vi "Analyze Data.vi"(0 "Weather Data":dynamicdata(waveform), 11 "error in":errorcluster) -> (4 "Time":dbl, 6 "Temperature":dbl, 8 "Wind Speed":dbl, 15 "error out":errorcluster)   [LabVIEW 2010]
uses:
  Instance           1 20Saved   Analyze Data .vi
  Instance           3 20Saved   Analyze Data .vi
  Instance           4 20Saved   Analyze Data .vi
  Instance           5 20Saved   Analyze Data .vi
  Instance           2 20Saved   Analyze Data .vi
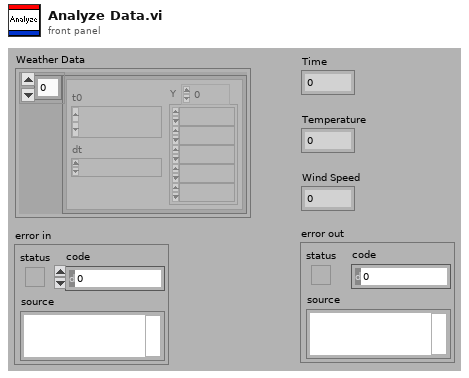
[diagram p1: front panel]
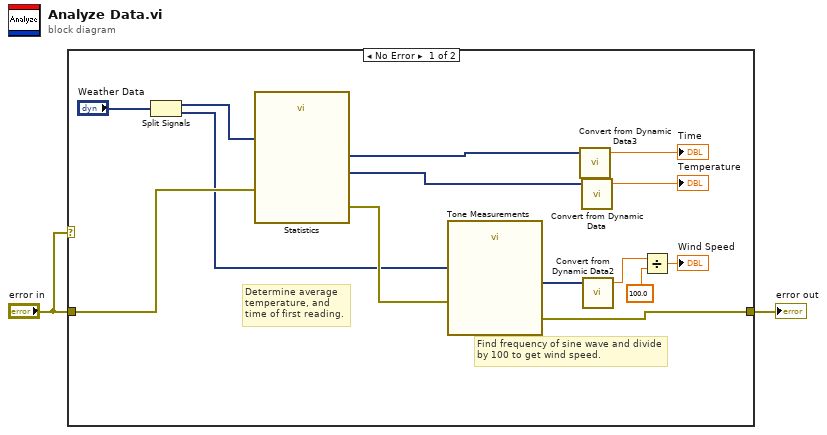
[diagram p0: block diagram]
diagram:
  n1 = case shown="No Error" "error in" {
    tunnel: "error in" -> [w16 w17]
    tunnel: [w10 w17] -> w2
    frame No Error {
      # "Find frequency of sine wave and divide by 100 to get wind speed."
      # "Determine average temperature, and time of first reading."
      n2 = Split Signals("Weather Data") -> (w4:dynamicdata, w3:dynamicdata)  [unwired: 2 in]
      n3 = call "Statistics"("Signals"=w4, "error in (no error)"=w16) -> ("Arithmetic Mean"=w5:dynamicdata, "First Time"=w11:dynamicdata, "error out"=w9:errorcluster)  [unwired: 23 in]
      n4 = call "Tone Measurements"("error in (no error)"=w9, "Signals"=w3) -> ("error out"=w10:errorcluster, "Frequency"=w7:dynamicdata)  [unwired: 8 in]
      n5 = call "Convert from Dynamic Data3"("Dynamic Data Type"=w11) -> ("Scalar"=→"Time":dbl)  [unwired: 3 in]
      n6 = call "Convert from Dynamic Data"("Dynamic Data Type"=w5) -> ("Scalar"=→"Temperature":dbl)  [unwired: 3 in]
      n7 = call "Convert from Dynamic Data2"("Dynamic Data Type"=w7) -> ("Scalar"=w8:dbl)  [unwired: 3 in]
      n8 = Divide(x=w8, y=100.0) -> (x/y=→"Wind Speed":dbl)
    }
    frame Error {
    }
  }
  "error out" <- w2
